vi "Auto_Init.vi"(5 "Wheel Arm Up":u8, 7 "Second Goal Init":u8, 8 "IR Pivot Left":u8, 9 "Goal Down":u8, 10 "Dump Up":u8, 11 "IR Arm Down":u8) -> (3 "BrickReference out":T1)   [LabVIEW 2012, in "Serenity_mk2.lvrbt"]
uses:
  Serenity_mk2.lvrbt
  <vilib>/NXT/Subs/LVHSConnector.ctl
  <vilib>/NXT/LegoClasses/BrickReference/BrickReference.lvclass
  <vilib>/NXT/Hardware/Plugins/Tetrix DC Motor/TetrixDCMotorAddress.ctl
  <vilib>/NXT/Hardware/Plugins/Tetrix 180 deg Servo/Tetrix180ServoAddress.ctl
  <vilib>/NXT/NXTIO Xnodes/NXTIONodeSubVIs/TETRIX IO Check Battery.vi
  <vilib>/NXT/NXTIO Xnodes/NXTIONodeSubVIs/TETRIX IO Move Servos.vi
  <vilib>/NXT/NXTIO Xnodes/NXTIONodeSubVIs/TETRIX IO Reset Encoders.vi
  <vilib>/NXT/NXTIO Xnodes/AddressXNode/NXTIOAddress.xnode
  <vilib>/NXT/NXTIO Xnodes/NXTIOXNode/NXTIO.xnode
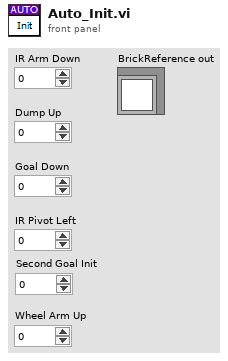
[diagram p1: front panel]
types:
  T1 = typedef "LVHSConnector.ctl" = refnum<class "BrickReference.lvclass">
  T2 = typedef "TetrixDCMotorAddress.ctl" = i32
  T3 = typedef "Tetrix180ServoAddress.ctl" = i32
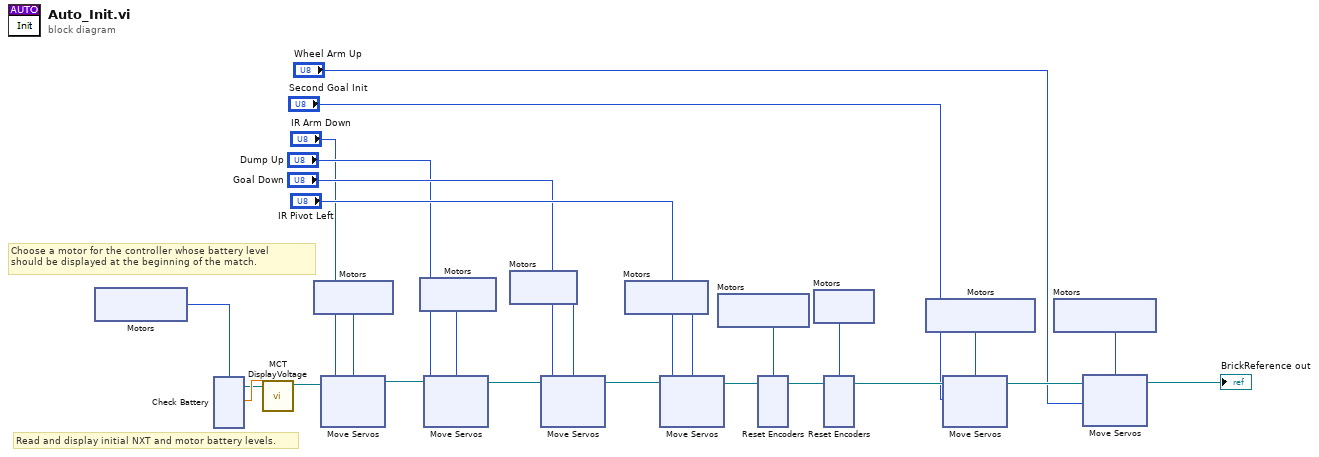
[diagram p0: block diagram]
diagram:
  # "Read and display initial NXT and motor battery levels."
  # "Choose a motor for the controller whose battery level \nshould be displayed at the beginning of the match."
  n1 = xnode "Motors"() -> ("Motor"=w10:T2)
  n2 = xnode "Check Battery"("Motors"=w10) -> ("Voltage 1"=w9:sgl, "NXT/EV3"=w8:T1)  [unwired: 1 in]
  n3 = call <vilib>:"MCT DisplayVoltage.vi"("Motor Voltage"=w9, "NXT"=w8) -> ("NXT"=w26:T1)  [unwired: 9 in]
  n4 = xnode "Motors"() -> ("Motor"=w12:T3)
  n5 = xnode "Move Servos"("Position 1"="IR Arm Down", "Motors"=w12, "NXT/EV3"=w26) -> ("NXT/EV3"=w13:T1)
  n6 = xnode "Motors"() -> ("Motor"=w25:T3)
  n7 = xnode "Move Servos"("Position 1"="Dump Up", "Motors"=w25, "NXT/EV3"=w13) -> ("NXT/EV3"=w14:T1)
  n8 = xnode "Motors"() -> ("Motor"=w17:T3)
  n9 = xnode "Move Servos"("Position 1"="Goal Down", "Motors"=w17, "NXT/EV3"=w14) -> ("NXT/EV3"=w15:T1)
  n10 = xnode "Motors"() -> ("Motor"=w19:T3)
  n11 = xnode "Move Servos"("Position 1"="IR Pivot Left", "Motors"=w19, "NXT/EV3"=w15) -> ("NXT/EV3"=w22:T1)
  n12 = xnode "Motors"() -> ("Motor"=w21:T2)
  n13 = xnode "Reset Encoders"("Motors"=w21, "NXT/EV3"=w22) -> ("NXT/EV3"=w24:T1)
  n14 = xnode "Motors"() -> ("Motor"=w23:T2)
  n15 = xnode "Reset Encoders"("Motors"=w23, "NXT/EV3"=w24) -> ("NXT/EV3"=w7:T1)
  n16 = xnode "Motors"() -> ("Motor"=w6:T3)
  n17 = xnode "Move Servos"("Position 1"="Second Goal Init", "Motors"=w6, "NXT/EV3"=w7) -> ("NXT/EV3"=w3:T1)
  n18 = xnode "Motors"() -> ("Motor"=w4:T3)
  n19 = xnode "Move Servos"("Position 1"="Wheel Arm Up", "Motors"=w4, "NXT/EV3"=w3) -> ("NXT/EV3"=→"BrickReference out":T1)
